vi "Send Message.vi"(6 "Timeout (5000)":i32=5000, 8 "error in (no error)":errorcluster, 10 "Message":string, 11 "0MQ_Server in":refnum<class "0MQ_Server.lvclass">) -> (0 "error out":errorcluster, 1 "Timeout?":bool, 2 "Reply Message (if waiting)":cluster{"identity":string, "data":string[]}, 3 "0MQ_Server out":refnum<class "0MQ_Server.lvclass">)   [LabVIEW 2016, in "0MQ_Server.lvclass"]
uses:
  0MQ_Server.lvclass
  0MQ_Server.lvclass/0MQ_Server.ctl
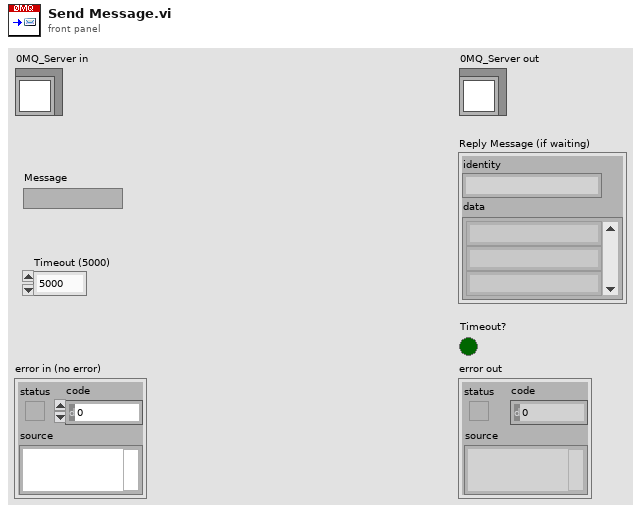
[diagram p1: front panel]
types:
  T1 = typedef "zeromq.lvlib/socket_type.ctl" = enum8{"ZMQ_PAIR", "ZMQ_PUB", "ZMQ_SUB", "ZMQ_REQ", "ZMQ_REP", "ZMQ_DEALER", "ZMQ_ROUTER", "ZMQ_PULL", "ZMQ_PUSH", "ZMQ_XPUB", "ZMQ_XSUB"}
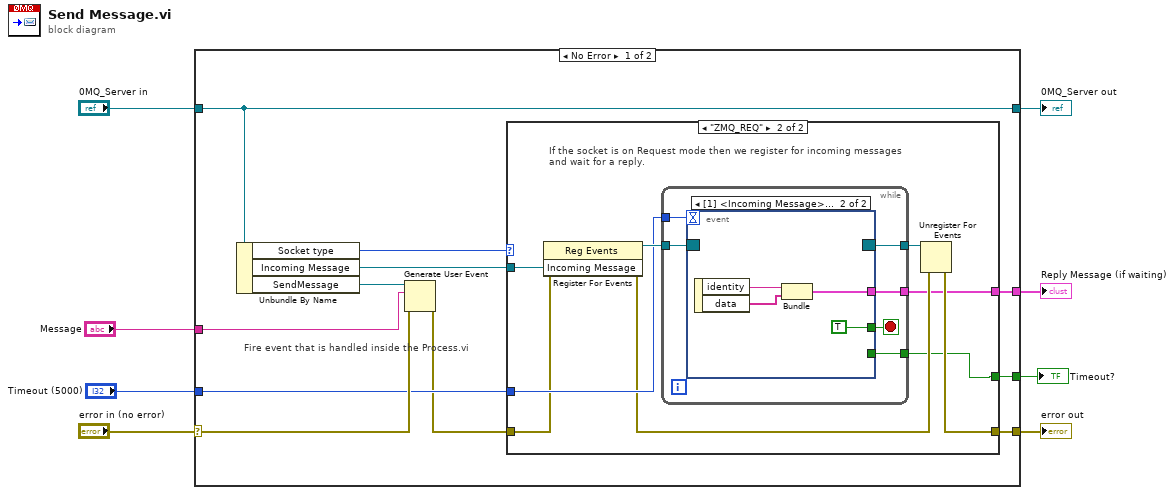
[diagram p0: block diagram]
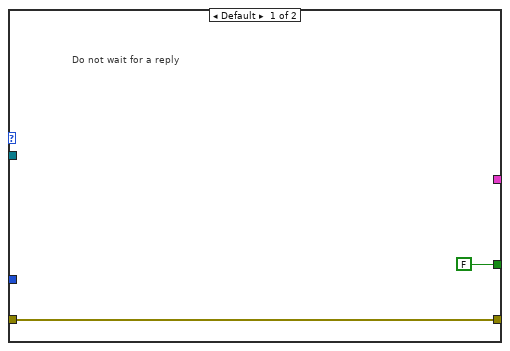
[diagram p2: hidden frame]
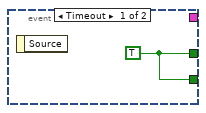
[diagram p3: hidden frame]
diagram:
  n1 = case shown="No Error" "error in (no error)" {
    selector: "error in (no error)" -> [w18 w43]
    tunnel: [w13 w43] -> w7
    tunnel: [w19 w42] -> w5
    tunnel: "0MQ_Server in" -> [w19 w42]
    tunnel: "Message" -> [w16 _]
    tunnel: "Timeout (5000)" -> [w14 _]
    tunnel: [w10 _] -> w2
    tunnel: [w9 _] -> w1
    frame No Error {
      # "Fire event that is handled inside the Process.vi"
      n2 = Unbundle By Name(w19) -> ("Socket type"=w11:T1, "Incoming Message"=w15:refnum<user-event>, "SendMessage"=w17:refnum<user-event>)
      n3 = Generate User Event(user event=w17, event data cluster=w16, error in=w18) -> (error out=w12:errorcluster)  [unwired: 1 in, 1 out]
      n4 = case shown="\"ZMQ_REQ\"" w11 {
        tunnel: w15 -> [_ w30]
        tunnel: w14 -> [_ w28]
        tunnel: [w21 w24] -> w13
        tunnel: w12 -> [w21 w27]
        tunnel: [_ w23] -> w10
        tunnel: [FALSE w22] -> w9
        frame Default {
          # "Do not wait for a reply"
        }
        frame "ZMQ_REQ" {
          # "If the socket is on Request mode then we register for incoming messages\nand wait for a reply."
          n5 = register-events(error in=w27, w30) -> (reference out=w29:refnum<event-registration>, error out=w25:errorcluster)  [unwired: 1 in]
          n6 = while {
            tunnel: w29 -> [w36]
            tunnel: w28 -> [w35]
            tunnel: [w34] -> w26
            tunnel: [w32] -> w23
            tunnel: [w31] -> w22
            stop <- w33 stop-if-true
            n7 = event shown="[1] <Incoming Message>: User Event" {
              selector: w36 -> [_ _]
              dyn-events: [_ _] -> w34
              timeout: w35 -> [_ _]
              tunnel: [w37 TRUE] -> w33
              tunnel: [_ w38] -> w32
              tunnel: [w37 _] -> w31
              event Timeout {
                w37 = TRUE
                n8 = event-data() -> ()  [unwired: 1 in, 1 out]
              }
              event User Event {
                n9 = event-data() -> ("identity"=w40:string, "data"=w39:string[])  [unwired: 1 in]
                n10 = Bundle("identity"=w40, "data"=w39) -> (w38:cluster{"identity":string, "data":string[]})  [unwired: 1 in]
              }
            }
          }
          n11 = Unregister For Events(event registration refnum=w26, error in=w25) -> (error out=w24:errorcluster)
        }
      }
    }
    frame Error {
    }
  }
  "error out" <- w7
  "0MQ_Server out" <- w5
  "Reply Message (if waiting)" <- w2
  "Timeout?" <- w1
